vi "H2_Control.vi"() -> ()   [LabVIEW 2019]
uses:
  Pressure Control CTL/DevHandshake_elt.ctl
  Pressure Control CTL/DevHandshake.ctl
  <instrlib>/Bronkhorst FLOW-BUS/Public/Configure/Setpoint/Configure Setpoint (Percentage).vi
  <instrlib>/Bronkhorst FLOW-BUS/Public/Data/Measure/Read Measure (Percentage).vi
  <instrlib>/Bronkhorst FLOW-BUS/Public/Data/Setpoint/Read Setpoint (Direct).vi
  <instrlib>/Bronkhorst FLOW-BUS/Public/Configure/Setpoint/Configure Setpoint (Direct).vi
  <instrlib>/Bronkhorst FLOW-BUS/Public/Data/Measure/Read Measure (Direct).vi
  <instrlib>/Bronkhorst FLOW-BUS/Bronkhorst FLOW-BUS.lvlib
panel:
  out "Initalised ?":bool
  out "Temperature (°C)":sgl
  out "Orifice Size (mm)":sgl
  in  "Read All":bool
  in  "Gas Type":u32(ring) items=["N2"=78, "He"=54, "H2"=56, "Ar"=5]
  out "Mass Flow":sgl
  out "Full Scale (bar a)":dbl
  in  "Change setpoint":bool
  out "Current pressure status":string
  in  "Pressure tolerance (%)":dbl=2.0
  out "Outlet Pressure (bar a)":sgl
  in  "Pressure Setpoint":sgl
  out "Status":string
  in  "DevNum":i16
  in  "Dev ID":string
  in  "Lock to Network":bool
  in  "Capacity Unit":string
  in  "Stop":bool
  out "Error Out":errorcluster
  in  "Node":u8=3
  in  "Baud Rate":u32=38400
  in  "VISA resource name":refnum<visa-resource-name>="COM1"
  in  "Start":bool
  out "DevSave":T1
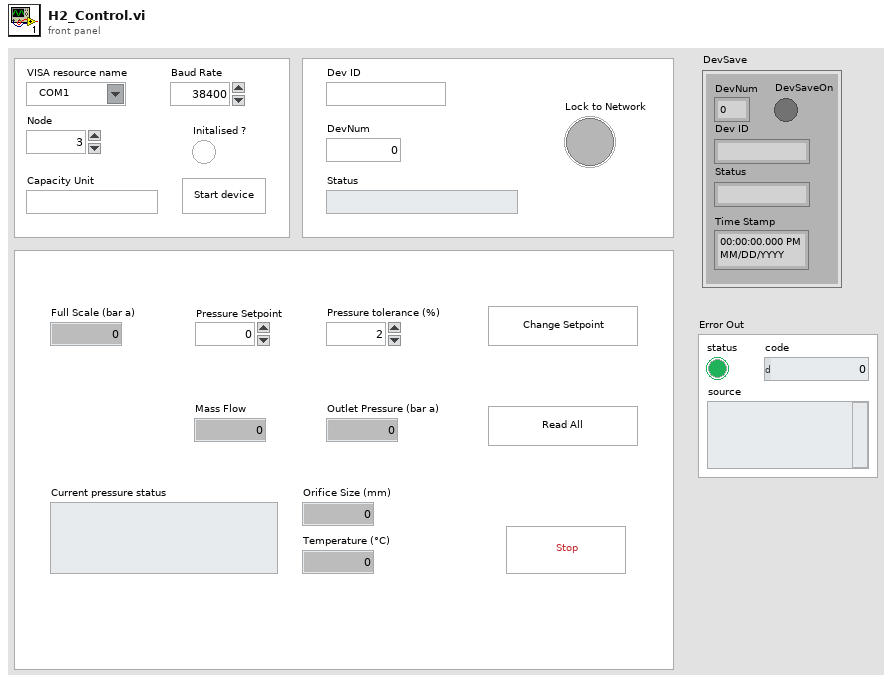
[diagram p1: front panel]
types:
  T1 = typedef "DevHandshake_elt.ctl" = cluster{"DevSaveOn":bool, "DevNum":i16, "Dev ID":string, "Status":string, "Time Stamp":timestamp}
  T2 = typedef "DevHandshake.ctl" = cluster{"DevSaveOn":bool, "DevNum":i16, "Dev ID":string, "Status":string, "Time Stamp":timestamp}[]
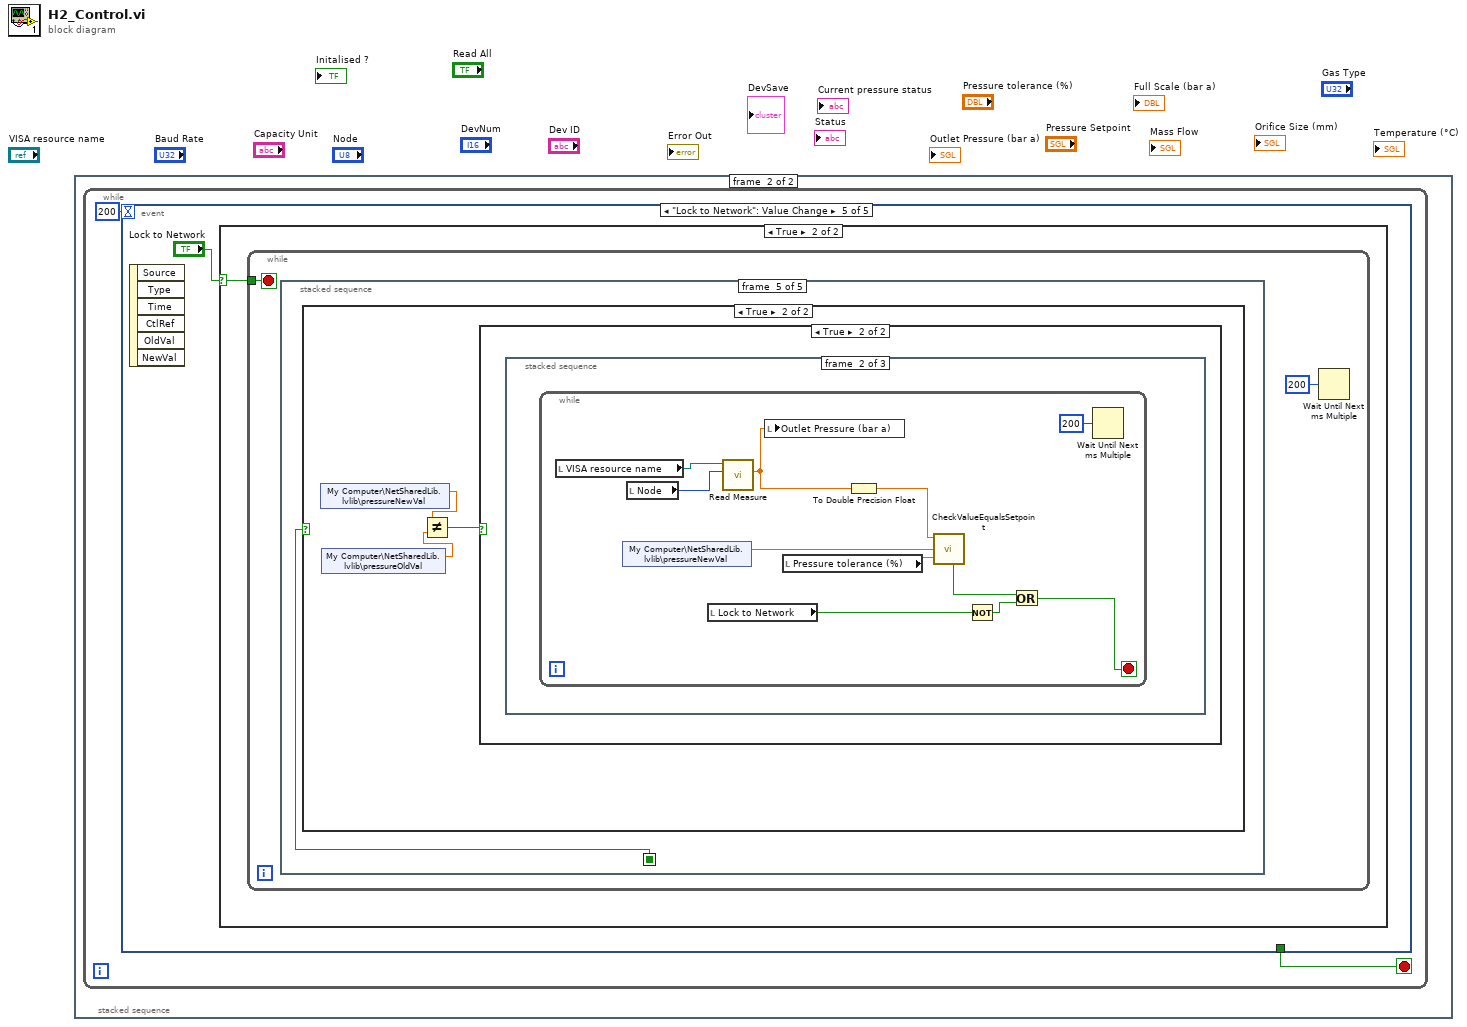
[diagram p0: block diagram]
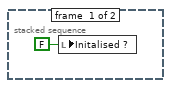
[diagram p2: hidden frame]
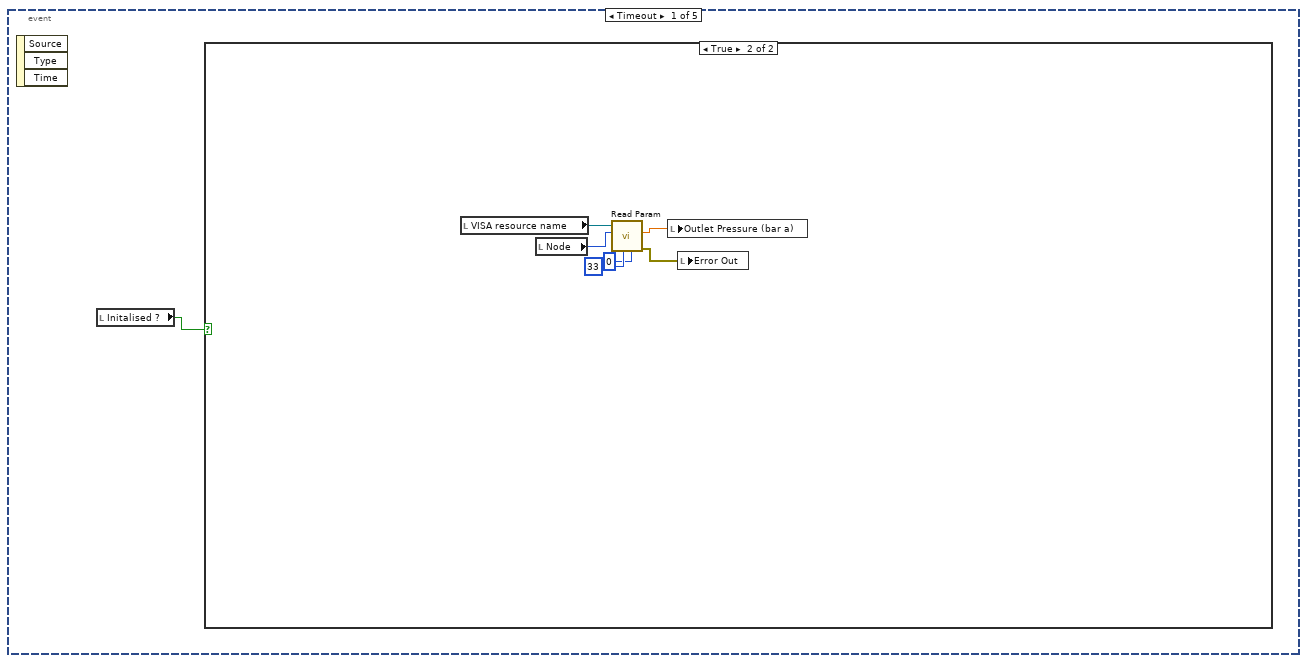
[diagram p3: hidden frame]
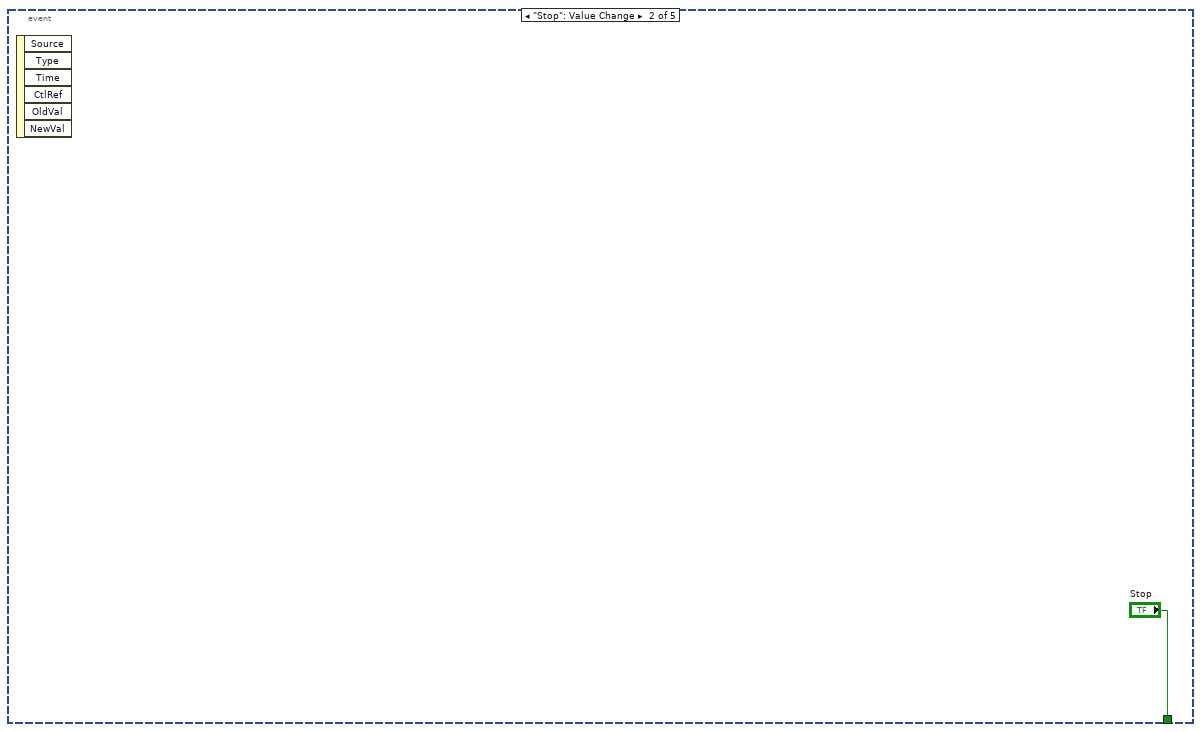
[diagram p5: hidden frame]
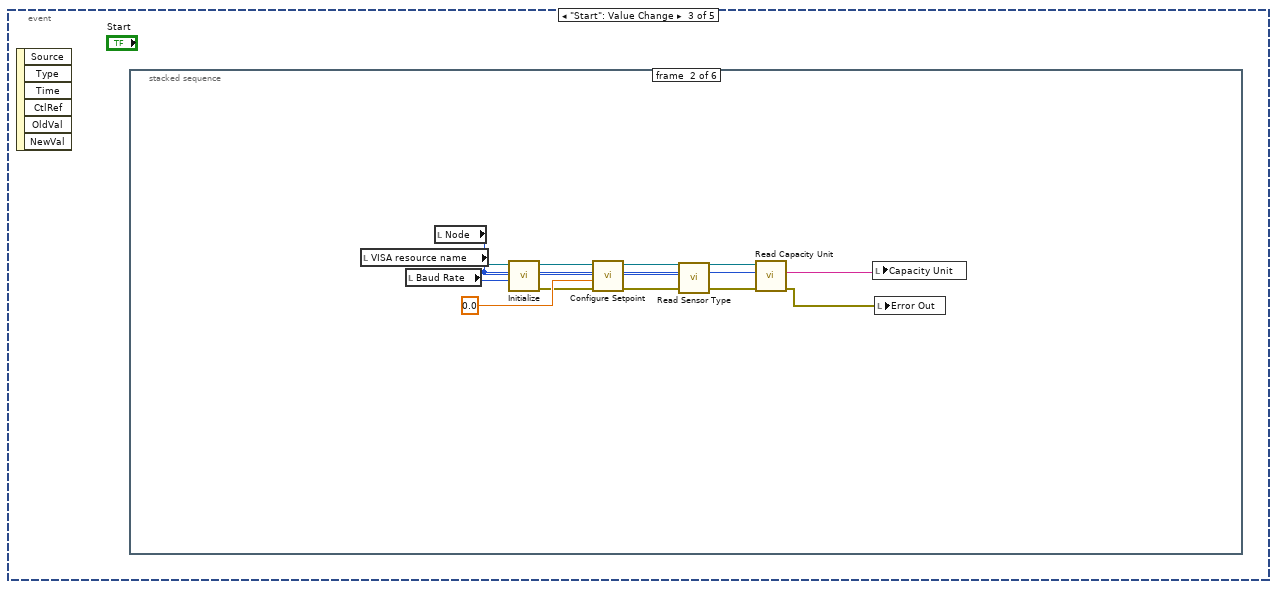
[diagram p6: hidden frame]
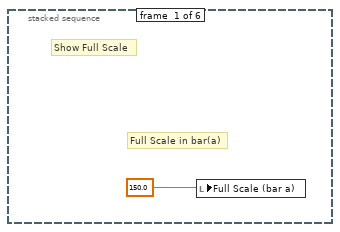
[diagram p7: hidden frame]
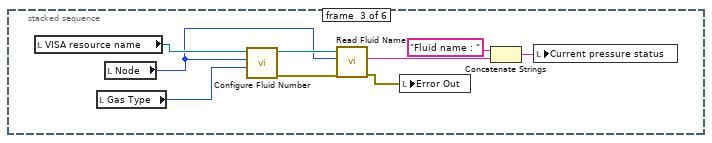
[diagram p8: hidden frame]
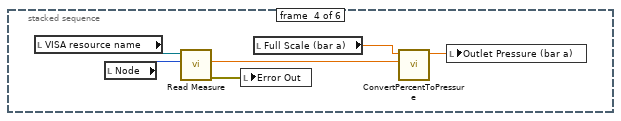
[diagram p9: hidden frame]
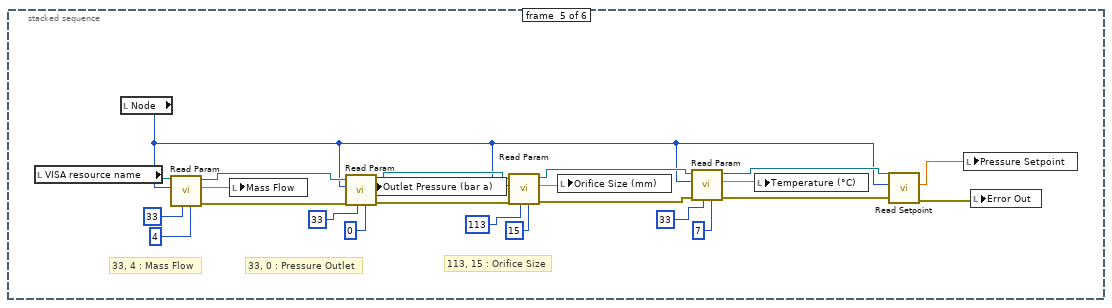
[diagram p10: hidden frame]
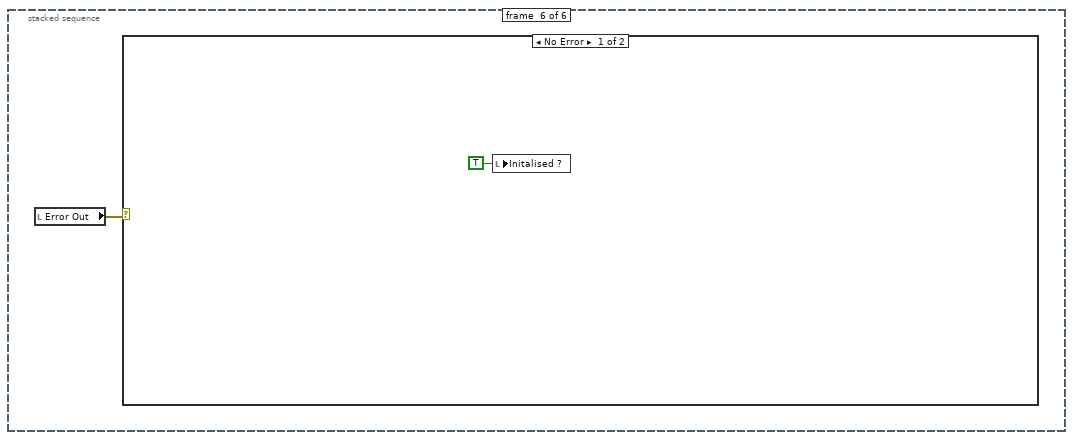
[diagram p11: hidden frame]
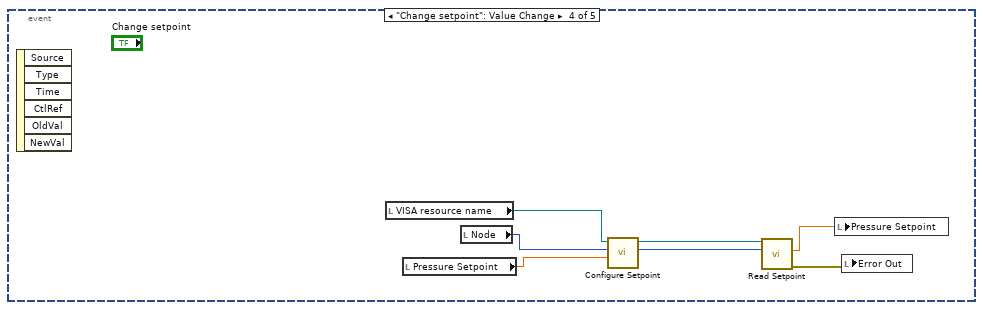
[diagram p13: hidden frame]
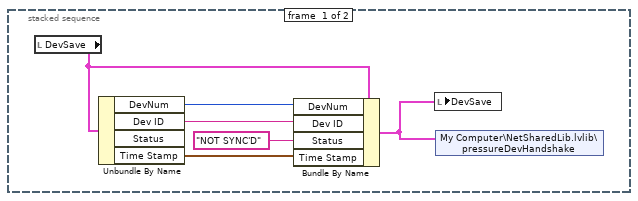
[diagram p15: hidden frame]
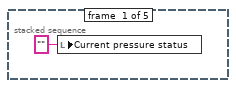
[diagram p16: hidden frame]
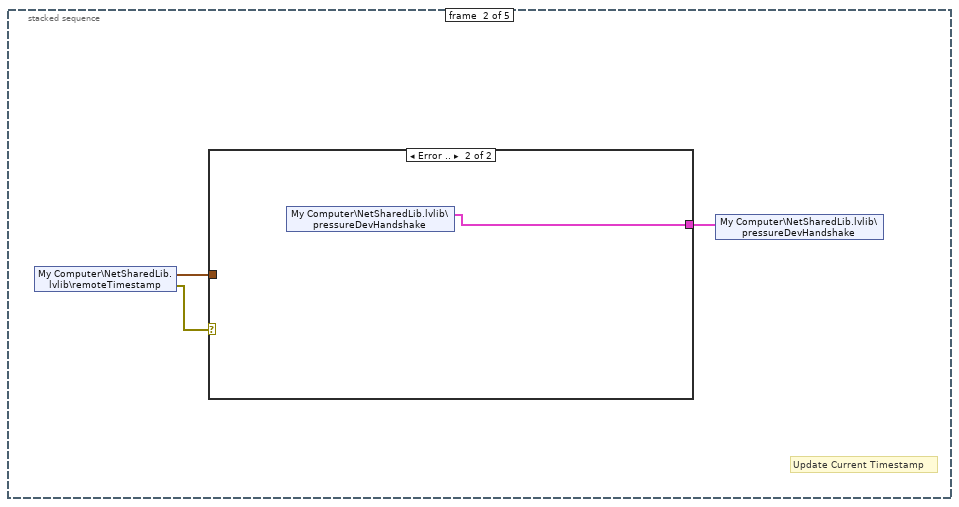
[diagram p17: hidden frame]
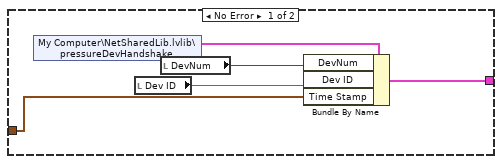
[diagram p18: hidden frame]
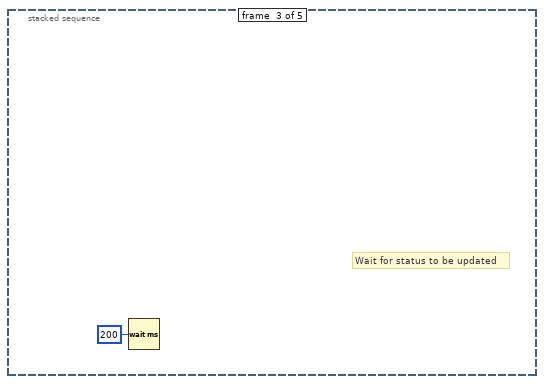
[diagram p19: hidden frame]
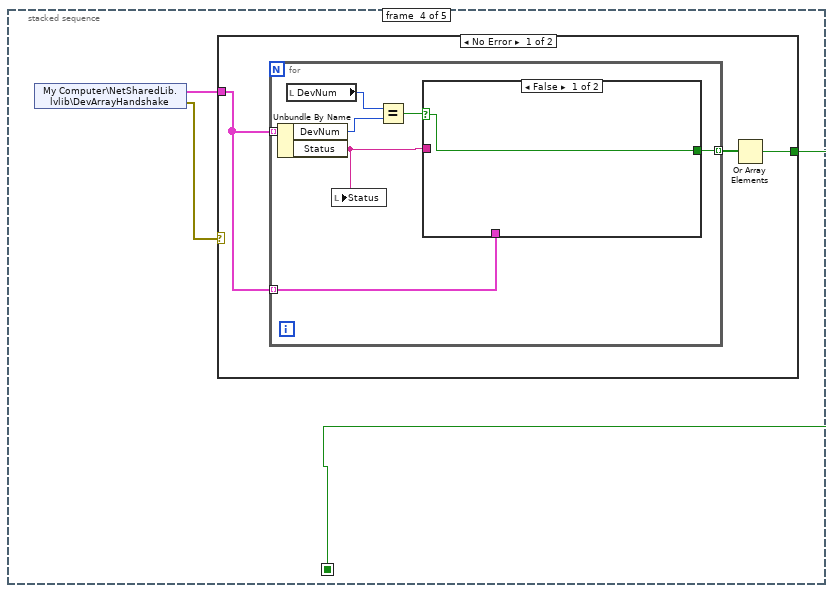
[diagram p20: hidden frame]
diagram:
  n1 = stacked-sequence {
    frame #0 {
      n2 = local write "Initalised ?"(FALSE ("Initalised ?")) -> ()
    }
    frame #1 {
      n3 = while {
        stop <- w3 stop-if-true
        n4 = event shown="[4] \"Lock to Network\": Value Change" {
          selector: _ -> [_ _ _ _ _]
          dyn-events: _ -> [_ _ _ _ _]
          timeout: 200 -> [_ _ _ _ _]
          tunnel: [_ "Stop" _ _ _] -> w3
          event Timeout {
            n5 = event-data() -> ()  [unwired: 1 in, 3 out]
            n6 = local read "Initalised ?"() -> (w4:bool)
            n7 = case shown="True" w4 {
              frame False {
              }
              frame True {
                n8 = local read "VISA resource name"() -> (w10:refnum<visa-resource-name>)
                n9 = local read "Node"() -> (w9:u8)
                n10 = call <instrlib>:"Read Param.vi"("Parameter (0)"=u16 0, "Process (0)"=u16 33, "Node (3)"=w9, "VISA resource name"=w10) -> ("error out"=w5:errorcluster, "Parameter Value"=w6:sgl)  [unwired: 5 in, 1 out]
                n11 = local write "Outlet Pressure (bar a)"(w6) -> ()
                n12 = local write "Error Out"(w5) -> ()
              }
            }
          }
          event "Stop": Value Change {
            n13 = event-data() -> ()  [unwired: 1 in, 6 out]
          }
          event "Start": Value Change {
            n14 = event-data() -> ()  [unwired: 1 in, 6 out]
            n15 = stacked-sequence {
              frame #0 {
                # "Full Scale in bar(a)"
                # "Show Full Scale"
                n16 = local write "Full Scale (bar a)"(150.0) -> ()
              }
              frame #1 {
                n17 = local read "VISA resource name"() -> (w24:refnum<visa-resource-name>)
                n18 = local read "Baud Rate"() -> (w23:u32)
                n19 = local read "Node"() -> (w16:u8)
                n20 = call <instrlib>:"Initialize.vi"("Baud Rate (38400)"=w23, "Node (3)"=w16, "VISA resource name"=w24) -> ("error out"=w20:errorcluster, "VISA resource name out"=w22:refnum<visa-resource-name>)  [unwired: 7 in]
                n21 = call-poly <instrlib>:"Configure Setpoint.vi"("error in (no error)"=w20, "Setpoint Percentage (0%)"=0.0, "Node (3)"=w16, "VISA resource name"=w22) -> ("error out"=w18:errorcluster, "VISA resource name out"=w19:refnum<visa-resource-name>)  [unwired: 6 in]
                n22 = call <instrlib>:"Read Sensor Type.vi"("error in (no error)"=w18, "Node (3)"=w16, "VISA resource name"=w19) -> ("error out"=w15:errorcluster, "VISA resource name out"=w17:refnum<visa-resource-name>)  [unwired: 5 in, 2 out]
                n23 = call <instrlib>:"Read Capacity Unit.vi"("error in (no error)"=w15, "Node (3)"=w16, "VISA resource name"=w17) -> ("error out"=w14:errorcluster, "Capacity Unit"=w13:string)  [unwired: 6 in, 1 out]
                n24 = local write "Capacity Unit"(w13) -> ()
                n25 = local write "Error Out"(w14) -> ()
              }
              frame #2 {
                n26 = local read "VISA resource name"() -> (w33:refnum<visa-resource-name>)
                n27 = local read "Gas Type"() -> (w32:u32)
                n28 = local read "Node"() -> (w30:u8)
                n29 = call <instrlib>:"Configure Fluid Number.vi"("Fluid Number (0)"=w32, "Node (3)"=w30, "VISA resource name"=w33) -> ("error out"=w29:errorcluster, "VISA resource name out"=w31:refnum<visa-resource-name>)  [unwired: 7 in]
                n30 = call <instrlib>:"Read Fluid Name.vi"("error in (no error)"=w29, "Node (3)"=w30, "VISA resource name"=w31) -> ("error out"=w25:errorcluster, "Fluid Name"=w27:string)  [unwired: 6 in, 1 out]
                n31 = local write "Error Out"(w25) -> ()
                n32 = Concatenate Strings("Fluid name : ", w27) -> (w26:string)
                n33 = local write "Current pressure status"(w26) -> ()
              }
              frame #3 {
                n34 = local read "VISA resource name"() -> (w37:refnum<visa-resource-name>)
                n35 = local read "Node"() -> (w36:u8)
                n36 = call-poly <instrlib>:"Read Measure.vi"("Node (3)"=w36, "VISA resource name"=w37) -> ("error out"=w34:errorcluster, "Measure Percentage"=w39:dbl)  [unwired: 7 in, 1 out]
                n37 = local write "Error Out"(w34) -> ()
                n38 = local read "Full Scale (bar a)"() -> (w35:dbl)
                n39 = call "ConvertPercentToPressure.vi"("Measure Percentage"=w39, "Full Scale (bar a)"=w35) -> ("Pressure (bar a)"=w38:dbl)  [unwired: 9 in]
                n40 = local write "Outlet Pressure (bar a)"(w38) -> ()
              }
              frame #4 {
                # "113, 15 : Orifice Size"
                # "33, 0 : Pressure Outlet"
                # "33, 4 : Mass Flow"
                n41 = local read "VISA resource name"() -> (w62:refnum<visa-resource-name>)
                n42 = local read "Node"() -> (w43:u8)
                n43 = call <instrlib>:"Read Param.vi"("Parameter (0)"=u16 4, "Process (0)"=u16 33, "Node (3)"=w43, "VISA resource name"=w62) -> ("error out"=w59:errorcluster, "Parameter Value"=w61:sgl, "VISA resource name out"=w60:refnum<visa-resource-name>)  [unwired: 5 in]
                n44 = local write "Mass Flow"(w61) -> ()
                n45 = call <instrlib>:"Read Param.vi"("Parameter (0)"=u16 0, "Process (0)"=u16 33, "error in (no error)"=w59, "Node (3)"=w43, "VISA resource name"=w60) -> ("error out"=w56:errorcluster, "Parameter Value"=w57:sgl, "VISA resource name out"=w55:refnum<visa-resource-name>)  [unwired: 4 in]
                n46 = local write "Outlet Pressure (bar a)"(w57) -> ()
                n47 = call <instrlib>:"Read Param.vi"("Parameter (0)"=u16 15, "Process (0)"=u16 113, "error in (no error)"=w56, "Node (3)"=w43, "VISA resource name"=w55) -> ("error out"=w51:errorcluster, "Parameter Value"=w53:sgl, "VISA resource name out"=w52:refnum<visa-resource-name>)  [unwired: 4 in]
                n48 = local write "Orifice Size (mm)"(w53) -> ()
                n49 = call <instrlib>:"Read Param.vi"("Parameter (0)"=u16 7, "Process (0)"=u16 33, "error in (no error)"=w51, "Node (3)"=w43, "VISA resource name"=w52) -> ("error out"=w42:errorcluster, "Parameter Value"=w48:sgl, "VISA resource name out"=w44:refnum<visa-resource-name>)  [unwired: 4 in]
                n50 = local write "Temperature (°C)"(w48) -> ()
                n51 = call-poly <instrlib>:"Read Setpoint.vi"("error in (no error)"=w42, "Node (3)"=w43, "VISA resource name"=w44) -> ("error out"=w40:errorcluster, "Setpoint Direct"=w41:sgl)  [unwired: 6 in, 1 out]
                n52 = local write "Pressure Setpoint"(w41) -> ()
                n53 = local write "Error Out"(w40) -> ()
              }
              frame #5 {
                n54 = local read "Error Out"() -> (w64:errorcluster)
                n55 = case shown="No Error" w64 {
                  frame No Error {
                    n56 = local write "Initalised ?"(TRUE ("Initalised ?")) -> ()
                  }
                  frame Error {
                  }
                }
              }
            }
          }
          event "Change setpoint": Value Change {
            n57 = event-data() -> ()  [unwired: 1 in, 6 out]
            n58 = local read "VISA resource name"() -> (w71:refnum<visa-resource-name>)
            n59 = local read "Pressure Setpoint"() -> (w68:sgl)
            n60 = local read "Node"() -> (w69:u8)
            n61 = call-poly <instrlib>:"Configure Setpoint.vi"("Setpoint Direct (0)"=w68, "Node (3)"=w69, "VISA resource name"=w71) -> ("VISA resource name out"=w70:refnum<visa-resource-name>)  [unwired: 7 in, 1 out]
            n62 = call-poly <instrlib>:"Read Setpoint.vi"("Node (3)"=w69, "VISA resource name"=w70) -> ("error out"=w66:errorcluster, "Setpoint Direct"=w67:sgl)  [unwired: 7 in, 1 out]
            n63 = local write "Pressure Setpoint"(w67) -> ()
            n64 = local write "Error Out"(w66) -> ()
          }
          event "Lock to Network": Value Change {
            n65 = event-data() -> ()  [unwired: 1 in, 6 out]
            n66 = case shown="True" "Lock to Network" {
              selector: "Lock to Network" -> [_ w79]
              frame False {
                n67 = stacked-sequence {
                  frame #0 {
                    n68 = local read "DevSave"() -> (w78:T1)
                    n69 = Unbundle By Name(w78) -> ("DevNum"=w77:i16, "Dev ID"=w76:string, "Time Stamp"=w74:timestamp)  [unwired: 1 out]
                    n70 = Bundle By Name(cluster=w78, "DevNum"=w77, "Dev ID"=w76, "Status"="NOT SYNC'D", "Time Stamp"=w74) -> (w73:T1)
                    n71 = local write "DevSave"(w73) -> ()
                    n72 = shared-variable "My Computer\\NetSharedLib.lvlib\\pressureDevHandshake"(w73) -> ()  [unwired: 1 in, 1 out]
                  }
                  frame #1 {
                    # "Read Current pressure"
                  }
                }
              }
              frame True {
                n73 = while {
                  tunnel: w79 -> [w81]
                  stop <- w81 stop-if-true
                  n74 = stacked-sequence {
                    seq-local: [_ _ _ w93 _] -> [_ _ _ _ w113]
                    frame #0 {
                      n75 = local write "Current pressure status"("" ("Current pressure status")) -> ()
                    }
                    frame #1 {
                      # "Update Current Timestamp"
                      n76 = shared-variable "My Computer\\NetSharedLib.lvlib\\remoteTimestamp"() -> (w84:timestamp, error out=w85:errorcluster)  [unwired: 1 in]
                      n77 = case shown="Error .." w85 {
                        tunnel: w84 -> [w89 _]
                        tunnel: [w86 w91] -> w83
                        frame No Error {
                          n78 = shared-variable "My Computer\\NetSharedLib.lvlib\\pressureDevHandshake"() -> (w90:T1)  [unwired: 1 in, 1 out]
                          n79 = local read "Dev ID"() -> (w88:string)
                          n80 = local read "DevNum"() -> (w87:i16)
                          n81 = Bundle By Name(cluster=w90, "DevNum"=w87, "Dev ID"=w88, "Time Stamp"=w89) -> (w86:T1)
                        }
                        frame Error {
                          n82 = shared-variable "My Computer\\NetSharedLib.lvlib\\pressureDevHandshake"() -> (w91:T1)  [unwired: 1 in, 1 out]
                        }
                      }
                      n83 = shared-variable "My Computer\\NetSharedLib.lvlib\\pressureDevHandshake"(w83) -> ()  [unwired: 1 in, 1 out]
                    }
                    frame #2 {
                      # "Wait for status to be updated"
                      n84 = Wait (ms)(milliseconds to wait=u32 200) -> ()  [unwired: 1 out]
                    }
                    frame #3 {
                      n85 = shared-variable "My Computer\\NetSharedLib.lvlib\\DevArrayHandshake"() -> (w94:T2, error out=w95:errorcluster)  [unwired: 1 in]
                      n86 = case shown="No Error" w95 {
                        tunnel: w94 -> [w98 _]
                        tunnel: [w96 FALSE] -> w93
                        frame No Error {
                          n87 = for {
                            tunnel: w98 -> [w105] mode=indexing
                            tunnel: w98 -> [w100] mode=indexing
                            tunnel: [w99] -> w97 mode=indexing
                            n88 = Unbundle By Name(w105) -> ("DevNum"=w103:i16, "Status"=w101:string)
                            n89 = local read "DevNum"() -> (w104:i16)
                            n90 = local write "Status"(w101) -> ()
                            n91 = Equal?(x=w104, y=w103) -> (x = y?=w102:bool)
                            n92 = case shown="False" w102 {
                              selector: w102 -> [w106 _]
                              tunnel: w101 -> [_ w108]
                              tunnel: w100 -> [_ w110]
                              tunnel: [w106 w107] -> w99
                              frame False {
                              }
                              frame True {
                                n93 = local write "DevSave"(w110) -> ()
                                n94 = Equal?(x=w108, y="Sync'd") -> (x = y?=w107:bool)
                              }
                            }
                          }
                          n95 = Or Array Elements(Boolean array=w97) -> (logical OR=w96:bool)
                        }
                        frame Error {
                          n96 = local write "Status"("Master not responding" ("Status")) -> ()
                        }
                      }
                    }
                    frame #4 {
                      n97 = case shown="True" w113 {
                        frame False {
                        }
                        frame True {
                          n98 = shared-variable "My Computer\\NetSharedLib.lvlib\\pressureNewVal"() -> (w115:dbl)  [unwired: 1 in, 1 out]
                          n99 = shared-variable "My Computer\\NetSharedLib.lvlib\\pressureOldVal"() -> (w116:dbl)  [unwired: 1 in, 1 out]
                          n100 = Not Equal?(x=w115, y=w116) -> (x != y?=w114:bool)
                          n101 = case shown="True" w114 {
                            frame False {
                            }
                            frame True {
                              n102 = stacked-sequence {
                                frame #0 {
                                # "Write setpoint"
                                n103 = shared-variable "My Computer\\NetSharedLib.lvlib\\pressureNewVal"() -> (w117:dbl)  [unwired: 1 in, 1 out]
                                n104 = local read "VISA resource name"() -> (w123:refnum<visa-resource-name>)
                                n105 = local read "Node"() -> (w122:u8)
                                n106 = call <instrlib>:"Write Param.vi"("Parameter (0)"=u16 3, "Process (0)"=u16 33, "Data for Float (0)"=w117, "Node (3)"=w122, "VISA resource name"=w123) -> ("error out"=w121:errorcluster)  [unwired: 4 in, 2 out]
                                n107 = To Single Precision Float(number=w117) -> (single precision float=w118:sgl)
                                n108 = local write "Error Out"(w121) -> ()
                                n109 = local write "Pressure Setpoint"(w118) -> ()
                                n110 = shared-variable "My Computer\\NetSharedLib.lvlib\\pressureOldVal"(w117) -> ()  [unwired: 1 in, 1 out]
                                }
                                frame #1 {
                                n111 = while {
                                stop <- w129 stop-if-true
                                n112 = local read "VISA resource name"() -> (w127:refnum<visa-resource-name>)
                                n113 = shared-variable "My Computer\\NetSharedLib.lvlib\\pressureNewVal"() -> (w134:dbl)  [unwired: 1 in, 1 out]
                                n114 = local read "Node"() -> (w126:u8)
                                n115 = local read "Lock to Network"() -> (w132:bool)
                                n116 = call-poly <instrlib>:"Read Measure.vi"("Node (3)"=w126, "VISA resource name"=w127) -> ("Measure Direct"=w125:sgl)  [unwired: 7 in, 2 out]
                                n117 = local write "Outlet Pressure (bar a)"(w125) -> ()
                                n118 = local read "Pressure tolerance (%)"() -> (w133:dbl)
                                n119 = To Double Precision Float(number=w125) -> (double precision float=w124:dbl)
                                n120 = call "CheckValueEqualsSetpoint.vi"("Pressure tolerance %"=w133, "PressureNewVal"=w134, "Pressure"=w124) -> ("PeqPSet ?"=w130:bool)  [unwired: 6 in, 1 out]
                                n121 = Not(x=w132) -> (.not. x?=w131:bool)
                                n122 = Or(x=w130, y=w131) -> (x .or. y?=w129:bool)
                                n123 = Wait Until Next ms Multiple(millisecond multiple=u32 200) -> ()  [unwired: 1 out]
                                }
                                }
                                frame #2 {
                                n124 = local read "Lock to Network"() -> (w135:bool)
                                n125 = case shown="True" w135 {
                                frame False {
                                }
                                frame True {
                                n126 = local read "Current pressure status"() -> (w139:string)
                                n127 = Concatenate Strings(w139, "\r" ("string"), "Connection to network was unlocked by user  " ("string")) -> (w136:string)
                                n128 = local write "Current pressure status"(w136) -> ()
                                }
                                }
                                }
                              }
                            }
                          }
                        }
                      }
                    }
                  }
                  n129 = Wait Until Next ms Multiple(millisecond multiple=u32 200) -> ()  [unwired: 1 out]
                }
              }
            }
          }
        }
      }
    }
  }
